vi "RPC Version.vi"(8 "error in (no error)":errorcluster, 11 "Hello in":refnum<class "Hello.lvclass">) -> (0 "error out":errorcluster, 2 "RPC Version":i32, 3 "Hello out":refnum<class "Hello.lvclass">)   [LabVIEW 2020, in "obs-websocket.lvlib" / "Hello.lvclass"]
uses:
  Hello.lvclass
  Hello.lvclass/Hello.ctl
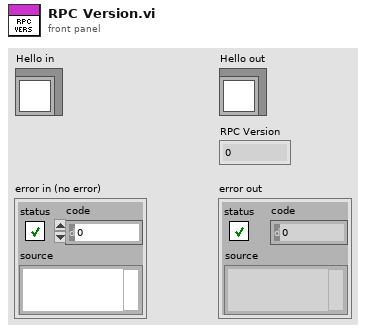
[diagram p1: front panel]
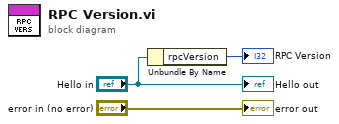
[diagram p0: block diagram]
diagram:
  n1 = Unbundle By Name("Hello in") -> ("rpcVersion"=→"RPC Version":i32)
  "error out" <- "error in (no error)"
  "Hello out" <- "Hello in"
